vi "RT Main v0.61.vi"() -> ()   [LabVIEW 2017]
uses:
  support/Controls/All Inputs.ctl
  support/Controls/Index Details.ctl
  Controls/Auto Delays.ctl
  Global Variables/RT GV.vi
  Global Variables/FPGA GV.vi
  <vilib>/Utility/error.llb/Error Cluster From Error Code.vi
  <vilib>/rvi/errors/niLvFpgaAdjustHostInterfaceError.vi
  Global Variables/Network Globals.vi
  support/Message Queue/Enqueue Message (Single).vi
  <vilib>/FPGAPlugInAG/Dynamic/niLvFpga_Close_Dynamic.vi
  <vilib>/rvi/interface/nirviReadWriteControl/nirviReadWriteControl.xnode
  Controls/FPGA Ref.ctl
  <vilib>/rvi/interface/nirviCloseFPGA/nirviCloseFPGA.xnode
  support/Message Queue/Message Queue.lvlib
  NiFpgaLv.dll
  <vilib>/rvi/interface/Simulation/niFpgaSimulationCallBeginRW.vi
panel:
  in  "Stop Button 2":bool
  out "Agitator Delays":u32[](array[numeric])=[400, 5000]
  out "error out":errorcluster
  out "Wrong Message":string
  in  "Stop Button":bool
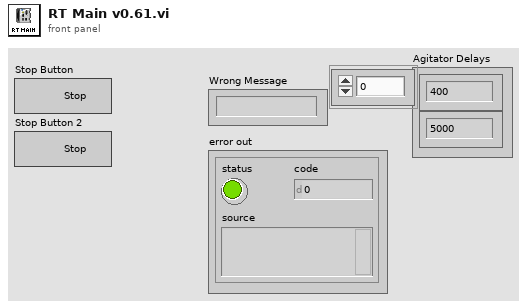
[diagram p1: front panel]
types:
  T1 = typedef "FPGA Ref.ctl" = refnum<k20>
  T2 = cluster{"TL_Red":bool, "TL_Orange":bool, "TL_Green":bool, "TL_Buzzer":bool, "SOL_Index_Rotary_CW":bool, "SOL_Index_CNVR_Rotary_CCW":bool, "SOL_Index_CNVR_Stopper_Rear":bool, "SOL_Index_CNVR_Output _Separator _Rear":bool, "Bowl  Feeder_ ON":bool, "Pump_CNVR_Motor _ON":bool, "SOL_Gating_CYL_Rear":bool, "SOL_Tube_Feed_Agitatator":bool, "SOL_Tube_Feed_Gating_CYL":bool, "SOL_Insertion _CYL":bool, "SOL_Insertion_Clamp_CYL":bool, "SOL_Cutting_CYL":bool, "SOL_Cutting_Clamp_CYL":bool, "SOL_Insertion_Air_Nozzle":bool, "SOL_Measurement_CYL":bool, "SOL_Measure_Clamp_CYL":bool, "SOL_Rejection CYL_1":bool, "SOL_Rejection CYL_2":bool, "SOL_Rejection CYL_3":bool, "SOL_Rejection CYL_4":bool, "DO1.24":bool, "DO1.25":bool, "DO1.26":bool, "DO1.27":bool, "DO1.28":bool, "DO1.29":bool, "DO1.30":bool, "DO1.31":bool}
  T3 = typedef "All Inputs.ctl" = cluster{"DI 1":cluster{"Machine_ON":bool, "E_stop ":bool, "SW_Pressure":bool, "SW_Start ":bool, "SW_Reset":bool, "SW_Stop":bool, "SW_Door":bool, "RS_Index_Rotary_CW":bool, "RS_Index_Rotary_CCW":bool, "RS_Index_Stopper _Rear":bool, "RS_Index_Output_Separator_Rear":bool, "PES_Index_Pallet_Sensor":bool, "PES_Index_Output_Part Sensor":bool, "ICS_BF_Low_Level_1":bool, "ICS_BF_Low_Level_2":bool, "ICS_BF_Pump_CNVR_Full_1":bool, "ICS_BF_Pump_CNVR_Full_2":bool, "ICS_BF_Pump_CNVR_Full_3":bool, "ICS_BF_Pump_CNVR_Full_4":bool, "PES_PC_Pump Presence_1":bool, "PES_PC_Pump Presence_2":bool, "PES_PC_Pump Presence_3":bool, "PES_PC_Pump Presence_4":bool, "RS_PC_Gating_Front":bool, "PES_Pump_Interference":bool, "PES_TF_Low_Level":bool, "PES_Tube Presence_1":bool, "PES_Tube Presence_2":bool, "PES_Tube Presence_3":bool, "PES_Tube Presence_4":bool, "DI1.30":bool, "DI1.31":bool}, "DI 2":cluster{"RS_Agitatator_1_Rear ":bool, "RS_Agitatator_2_Rear ":bool, "RS_TF_Gating CYL_Rear":bool, "RS_Insertion_1_Rear":bool, "RS_Insertion_1_Front":bool, "RS_Insertion _2_Rear":bool, "RS_Insertion _2_Front":bool, "RS_Insertion _3_Rear":bool, "RS_Insertion _3_Front":bool, "RS_Insertion _4_Rear":bool, "RS_Insertion _4_Front":bool, "RS_Insertion_Clamp_Rear":bool, "RS_Cutting_Rear":bool, "RS_Cutting_Clamp _Rear":bool, "RS_Measurement_1_Rear":bool, "RS_Measurement_2_Rear":bool, "RS_Measurement_3_Rear":bool, "RS_Measurement_4_Rear":bool, "RS_Measure_Clamp_Rear":bool, "RS_Rejection_1_Rear":bool, "RS_Rejection_2_Rear":bool, "RS_Rejection_3_Rear":bool, "RS_Rejection_4_Rear":bool, "DI2.23":bool, "DI2.24":bool, "DI2.25":bool, "DI2.26":bool, "DI2.27":bool, "DI2.28":bool, "DI2.29":bool, "DI2.30":bool, "DI2.31":bool}, "IAS 1":dbl, "IAS 2":dbl, "IAS 3":dbl, "IAS 4":dbl, "DO 1":cluster{"TL_Red":bool, "TL_Orange":bool, "TL_Green":bool, "TL_Buzzer":bool, "SOL_Index_Rotary_CW":bool, "SOL_Index_CNVR_Rotary_CCW":bool, "SOL_Index_CNVR_Stopper_Rear":bool, "SOL_Index_CNVR_Output _Separator _Rear":bool, "Bowl  Feeder_ ON":bool, "Pump_CNVR_Motor _ON":bool, "SOL_PC_Gating_CYL_Rear":bool, "SOL_Tube_Feed_Agitatator":bool, "SOL_Tube_Feed_Gating_CYL":bool, "SOL_Insertion _CYL":bool, "SOL_Insertion_Clamp_CYL":bool, "SOL_Cutting_CYL":bool, "SOL_Cutting_Clamp_CYL":bool, "SOL_Insertion_Air_Nozzle":bool, "SOL_Measurement_CYL":bool, "SOL_Measure_Clamp_CYL":bool, "SOL_Rejection CYL_1":bool, "SOL_Rejection CYL_2":bool, "SOL_Rejection CYL_3":bool, "SOL_Rejection CYL_4":bool, "DO1.24":bool, "DO1.25":bool, "DO1.26":bool, "DO1.27":bool, "DO1.28":bool, "DO1.29":bool, "DO1.30":bool, "DO1.31":bool}}
  T4 = typedef "Index Details.ctl" = cluster{"Time (ms)":u32, "Waveform Graph":i16[]}
  T5 = typedef "Auto Delays.ctl" = cluster{"Agitator Delays":u32[], "TF Delays":u32[], "Insertion Delays":u32[], "Cutting Delays":u32[], "PF Delays":u32[], "Measur. Delays":u32[], "Reject Delays":u32[]}
  T6 = cluster{T5, "Reject Pallets":cluster{"Reject 1":bool, "Reject 2":bool, "Reject 3":bool, "Reject 4":bool}}
  T7 = cluster{"TL_Red":bool, "TL_Orange":bool, "TL_Green":bool, "TL_Buzzer":bool, "SOL_Index_Rotary_CW":bool, "SOL_Index_CNVR_Rotary_CCW":bool, "SOL_Index_CNVR_Stopper_Rear":bool, "SOL_Index_CNVR_Output _Separator _Rear":bool, "Bowl  Feeder_ ON":bool, "Pump_CNVR_Motor _ON":bool, "SOL_PC_Gating_CYL_Rear":bool, "SOL_Tube_Feed_Agitatator":bool, "SOL_Tube_Feed_Gating_CYL":bool, "SOL_Insertion _CYL":bool, "SOL_Insertion_Clamp_CYL":bool, "SOL_Cutting_CYL":bool, "SOL_Cutting_Clamp_CYL":bool, "SOL_Insertion_Air_Nozzle":bool, "SOL_Measurement_CYL":bool, "SOL_Measure_Clamp_CYL":bool, "SOL_Rejection CYL_1":bool, "SOL_Rejection CYL_2":bool, "SOL_Rejection CYL_3":bool, "SOL_Rejection CYL_4":bool, "DO1.24":bool, "DO1.25":bool, "DO1.26":bool, "DO1.27":bool, "DO1.28":bool, "DO1.29":bool, "DO1.30":bool, "DO1.31":bool}
  T8 = cluster{"Machine_ON":bool, "E_stop ":bool, "SW_Pressure":bool, "SW_Start ":bool, "SW_Reset":bool, "SW_Stop":bool, "SW_Door":bool, "RS_Index_Rotary_CW":bool, "RS_Index_Rotary_CCW":bool, "RS_Index_Stopper _Rear":bool, "RS_Index_Output_Separator_Rear":bool, "PES_Index_Pallet_Sensor":bool, "PES_Index_Output_Part Sensor":bool, "ICS_BF_Low_Level_1":bool, "ICS_BF_Low_Level_2":bool, "ICS_BF_Pump_CNVR_Full_1":bool, "ICS_BF_Pump_CNVR_Full_2":bool, "ICS_BF_Pump_CNVR_Full_3":bool, "ICS_BF_Pump_CNVR_Full_4":bool, "PES_PC_Pump Presence_1":bool, "PES_PC_Pump Presence_2":bool, "PES_PC_Pump Presence_3":bool, "PES_PC_Pump Presence_4":bool, "RS_PC_Gating_Front":bool, "PES_Pump_Interference":bool, "PES_TF_Low_Level":bool, "PES_Tube Presence_1":bool, "PES_Tube Presence_2":bool, "PES_Tube Presence_3":bool, "PES_Tube Presence_4":bool, "DI1.30":bool, "DI1.31":bool}
  T9 = cluster{"RS_Agitatator_1_Rear ":bool, "RS_Agitatator_2_Rear ":bool, "RS_TF_Gating CYL_Rear":bool, "RS_Insertion_1_Rear":bool, "RS_Insertion_1_Front":bool, "RS_Insertion _2_Rear":bool, "RS_Insertion _2_Front":bool, "RS_Insertion _3_Rear":bool, "RS_Insertion _3_Front":bool, "RS_Insertion _4_Rear":bool, "RS_Insertion _4_Front":bool, "RS_Insertion_Clamp_Rear":bool, "RS_Cutting_Rear":bool, "RS_Cutting_Clamp _Rear":bool, "RS_Measurement_1_Rear":bool, "RS_Measurement_2_Rear":bool, "RS_Measurement_3_Rear":bool, "RS_Measurement_4_Rear":bool, "DI2.18":bool, "RS_Rejection_1_Rear":bool, "RS_Rejection_2_Rear":bool, "RS_Rejection_3_Rear":bool, "RS_Rejection_4_Rear":bool, "DI2.23":bool, "DI2.24":bool, "DI2.25":bool, "DI2.26":bool, "DI2.27":bool, "DI2.28":bool, "DI2.29":bool, "DI2.30":bool, "DI2.31":bool}
  T10 = cluster{"Reject 1":bool, "Reject 2":bool, "Reject 3":bool, "Reject 4":bool}
  T11 = typedef "Auto Times.ctl" = cluster{"Index Time":u32, "TF Time":u32, "Insertion Time":u32, "Cutting Time":u32, "PF Time":u32, "Meas. Time":u32, "Reject Time":u32}
  T12 = cluster{"Auto Times":T11, "Measurements":cluster{"1":dbl, "2":dbl, "3":dbl, "4":dbl}, "OutputCount":u32, "error out":errorcluster}
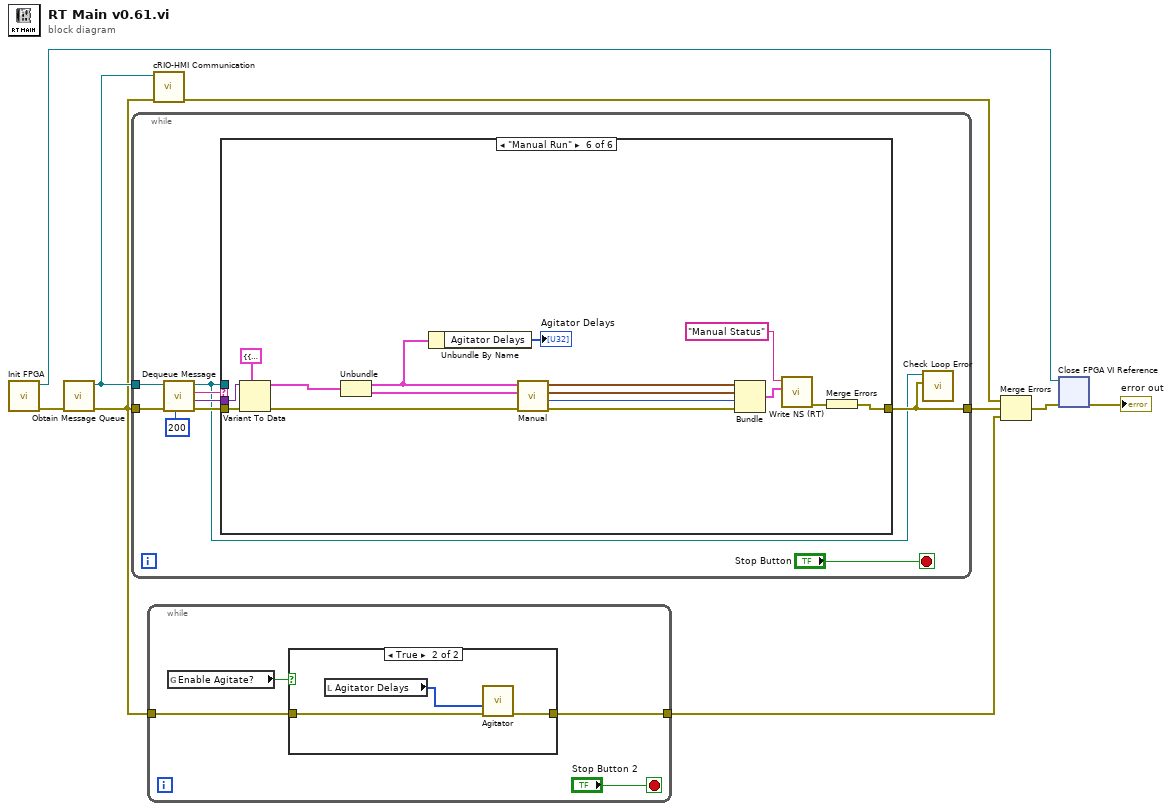
[diagram p0: block diagram]
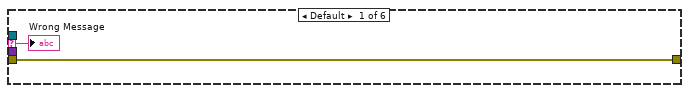
[diagram p3: hidden frame]
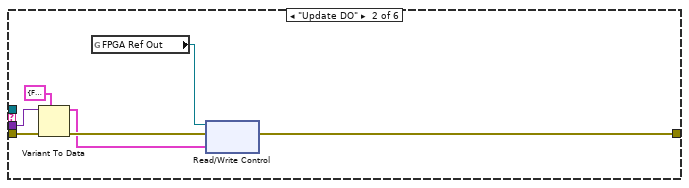
[diagram p4: hidden frame]
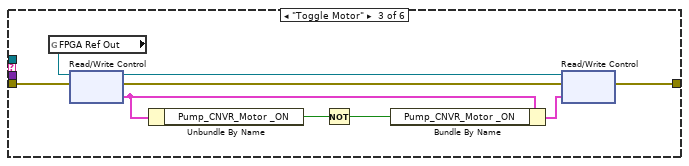
[diagram p5: hidden frame]
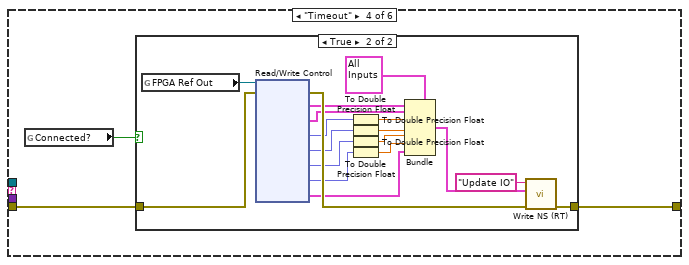
[diagram p6: hidden frame]
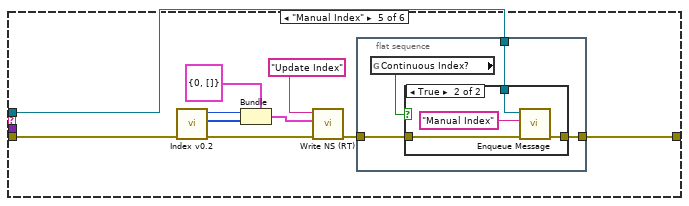
[diagram p8: hidden frame]
diagram:
  n1 = call "Init FPGA.vi"() -> ("error out"=w9:errorcluster, "FPGA Ref Out"=w3:T1)  [unwired: 10 in]
  n2 = call "Obtain Message Queue.vi"("error in (no error)"=w9) -> ("error out"=w2:errorcluster, "Message Queue"=w8:refnum<queue>)  [unwired: 9 in]
  n3 = while {
    tunnel: w2 -> [w17]
    tunnel: w8 -> [w16]
    tunnel: [w12] -> w7
    stop <- "Stop Button" stop-if-true
    n4 = call "Dequeue Message.vi"("timeout"=200, "error in (no error)"=w17, "Message Queue"=w16) -> ("error out"=w15:errorcluster, "Message Data"=w13:variant, "Message"=w14:string, "dup Message Queue"=w11:refnum<queue>)  [unwired: 5 in]
    n5 = case shown="\"Manual Run\"" w14 {
      selector: w14 -> [w20 _ _ _ _ _]
      tunnel: w15 -> [w19 w27 w35 w38 w68 w93]
      tunnel: w11 -> [_ _ _ _ w60 _]
      tunnel: w13 -> [_ w26 _ _ _ w92]
      tunnel: [w19 w22 w33 w39 w61 w88] -> w12
      frame Default {
        "Wrong Message" <- w20
      }
      frame "Update DO" {
        n6 = Variant To Data(error in=w27, type=T2 {"TL_Red"=FALSE, "TL_Orange"=FALSE, "TL_Green"=FALSE, "TL_Buzzer"=FALSE, "SOL_Index_Rotary_CW"=FALSE, "SOL_Index_CNVR_Rotary_CCW"=FALSE, "SOL_Index_CNVR_Stopper_Rear"=FALSE, "SOL_Index_CNVR_Output _Separator _Rear"=FALSE, "Bowl  Feeder_ ON"=FALSE, "Pump_CNVR_Motor _ON"=FALSE, "SOL_Gating_CYL_Rear"=FALSE, "SOL_Tube_Feed_Agitatator"=FALSE, "SOL_Tube_Feed_Gating_CYL"=FALSE, "SOL_Insertion _CYL"=FALSE, "SOL_Insertion_Clamp_CYL"=FALSE, "SOL_Cutting_CYL"=FALSE, "SOL_Cutting_Clamp_CYL"=FALSE, "SOL_Insertion_Air_Nozzle"=FALSE, "SOL_Measurement_CYL"=FALSE, "SOL_Measure_Clamp_CYL"=FALSE, "SOL_Rejection CYL_1"=FALSE, "SOL_Rejection CYL_2"=FALSE, "SOL_Rejection CYL_3"=FALSE, "SOL_Rejection CYL_4"=FALSE, "DO1.24"=FALSE, "DO1.25"=FALSE, "DO1.26"=FALSE, "DO1.27"=FALSE, "DO1.28"=FALSE, "DO1.29"=FALSE, "DO1.30"=FALSE, "DO1.31"=FALSE} ("DO 1"), Variant=w26) -> (data=w21:T2, error out=w23:errorcluster)
        n7 = global read "FPGA GV.vi" "FPGA Ref Out"() -> (w24:T1)
        n8 = xnode "Read/Write Control"("FPGA VI Reference In"=w24, "error in"=w23, "DO 1"=w21) -> ("error out"=w22:errorcluster)  [unwired: 1 out]
      }
      frame "Toggle Motor" {
        n9 = global read "FPGA GV.vi" "FPGA Ref Out"() -> (w36:T1)
        n10 = xnode "Read/Write Control"("FPGA VI Reference In"=w36, "error in"=w35) -> ("FPGA VI Reference Out"=w32:T1, "error out"=w34:errorcluster, "DO 1"=w30:T7)
        n11 = Unbundle By Name(w30) -> ("Pump_CNVR_Motor _ON"=w31:bool)
        n12 = Not(x=w31) -> (.not. x?=w28:bool)
        n13 = Bundle By Name(cluster=w30, "Pump_CNVR_Motor _ON"=w28) -> (w29:T7)
        n14 = xnode "Read/Write Control"("FPGA VI Reference In"=w32, "error in"=w34, "DO 1"=w29) -> ("error out"=w33:errorcluster)  [unwired: 1 out]
      }
      frame "Timeout" {
        n15 = global read "Network Globals.vi" "Connected?"() -> (w37:bool)
        n16 = case shown="True" w37 {
          tunnel: [w40 w57] -> w39
          tunnel: w38 -> [w40 w55]
          frame False {
          }
          frame True {
            n17 = global read "FPGA GV.vi" "FPGA Ref Out"() -> (w56:T1)
            n18 = xnode "Read/Write Control"("FPGA VI Reference In"=w56, "error in"=w55) -> ("error out"=w54:errorcluster, "DI 1"=w53:T8, "DI 2"=w52:T9, "AI0"=w51:fxp<+/-,27,6>, "AI1"=w46:fxp<+/-,27,6>, "AI2"=w45:fxp<+/-,27,6>, "AI3"=w44:fxp<+/-,27,6>, "DO 1"=w41:T7)  [unwired: 1 out]
            n19 = To Double Precision Float(number=w51) -> (double precision float=w50:dbl)
            n20 = To Double Precision Float(number=w46) -> (double precision float=w49:dbl)
            n21 = To Double Precision Float(number=w45) -> (double precision float=w48:dbl)
            n22 = To Double Precision Float(number=w44) -> (double precision float=w47:dbl)
            n23 = Bundle(cluster=T3 {"DI 1"={"Machine_ON"=FALSE, "E_stop "=FALSE, "SW_Pressure"=FALSE, "SW_Start "=FALSE, "SW_Reset"=FALSE, "SW_Stop"=FALSE, "SW_Door"=FALSE, "RS_Index_Rotary_CW"=FALSE, "RS_Index_Rotary_CCW"=FALSE, "RS_Index_Stopper _Rear"=FALSE, "RS_Index_Output_Separator_Rear"=FALSE, "PES_Index_Pallet_Sensor"=FALSE, "PES_Index_Output_Part Sensor"=FALSE, "ICS_BF_Low_Level_1"=FALSE, "ICS_BF_Low_Level_2"=FALSE, "ICS_BF_Pump_CNVR_Full_1"=FALSE, "ICS_BF_Pump_CNVR_Full_2"=FALSE, "ICS_BF_Pump_CNVR_Full_3"=FALSE, "ICS_BF_Pump_CNVR_Full_4"=FALSE, "PES_PC_Pump Presence_1"=FALSE, "PES_PC_Pump Presence_2"=FALSE, "PES_PC_Pump Presence_3"=FALSE, "PES_PC_Pump Presence_4"=FALSE, "RS_PC_Gating_Front"=FALSE, "PES_Pump_Interference"=FALSE, "PES_TF_Low_Level"=FALSE, "PES_Tube Presence_1"=FALSE, "PES_Tube Presence_2"=FALSE, "PES_Tube Presence_3"=FALSE, "PES_Tube Presence_4"=FALSE, "DI1.30"=FALSE, "DI1.31"=FALSE}, "DI 2"={"RS_Agitatator_1_Rear "=FALSE, "RS_Agitatator_2_Rear "=FALSE, "RS_TF_Gating CYL_Rear"=FALSE, "RS_Insertion_1_Rear"=FALSE, "RS_Insertion_1_Front"=FALSE, "RS_Insertion _2_Rear"=FALSE, "RS_Insertion _2_Front"=FALSE, "RS_Insertion _3_Rear"=FALSE, "RS_Insertion _3_Front"=FALSE, "RS_Insertion _4_Rear"=FALSE, "RS_Insertion _4_Front"=FALSE, "RS_Insertion_Clamp_Rear"=FALSE, "RS_Cutting_Rear"=FALSE, "RS_Cutting_Clamp _Rear"=FALSE, "RS_Measurement_1_Rear"=FALSE, "RS_Measurement_2_Rear"=FALSE, "RS_Measurement_3_Rear"=FALSE, "RS_Measurement_4_Rear"=FALSE, "RS_Measure_Clamp_Rear"=FALSE, "RS_Rejection_1_Rear"=FALSE, "RS_Rejection_2_Rear"=FALSE, "RS_Rejection_3_Rear"=FALSE, "RS_Rejection_4_Rear"=FALSE, "DI2.23"=FALSE, "DI2.24"=FALSE, "DI2.25"=FALSE, "DI2.26"=FALSE, "DI2.27"=FALSE, "DI2.28"=FALSE, "DI2.29"=FALSE, "DI2.30"=FALSE, "DI2.31"=FALSE}, "IAS 1"=0.0, "IAS 2"=0.0, "IAS 3"=0.0, "IAS 4"=0.0, "DO 1"={"TL_Red"=FALSE, "TL_Orange"=FALSE, "TL_Green"=FALSE, "TL_Buzzer"=FALSE, "SOL_Index_Rotary_CW"=FALSE, "SOL_Index_CNVR_Rotary_CCW"=FALSE, "SOL_Index_CNVR_Stopper_Rear"=FALSE, "SOL_Index_CNVR_Output _Separator _Rear"=FALSE, "Bowl  Feeder_ ON"=FALSE, "Pump_CNVR_Motor _ON"=FALSE, "SOL_PC_Gating_CYL_Rear"=FALSE, "SOL_Tube_Feed_Agitatator"=FALSE, "SOL_Tube_Feed_Gating_CYL"=FALSE, "SOL_Insertion _CYL"=FALSE, "SOL_Insertion_Clamp_CYL"=FALSE, "SOL_Cutting_CYL"=FALSE, "SOL_Cutting_Clamp_CYL"=FALSE, "SOL_Insertion_Air_Nozzle"=FALSE, "SOL_Measurement_CYL"=FALSE, "SOL_Measure_Clamp_CYL"=FALSE, "SOL_Rejection CYL_1"=FALSE, "SOL_Rejection CYL_2"=FALSE, "SOL_Rejection CYL_3"=FALSE, "SOL_Rejection CYL_4"=FALSE, "DO1.24"=FALSE, "DO1.25"=FALSE, "DO1.26"=FALSE, "DO1.27"=FALSE, "DO1.28"=FALSE, "DO1.29"=FALSE, "DO1.30"=FALSE, "DO1.31"=FALSE}}, "DI 1"=w53, "DI 2"=w52, "IAS 1"=w50, "IAS 2"=w49, "IAS 3"=w48, "IAS 4"=w47, "DO 1"=w41) -> (w43:T3)
            n24 = call "Write NS (RT).vi"("error in (no error)"=w54, "Message Data"=w43, "Message"="Update IO") -> ("error out"=w57:errorcluster)  [unwired: 8 in]
          }
        }
      }
      frame "Manual Index" {
        n25 = call "Index v0.2.vi"("error in (no error)"=w68) -> ("error out"=w66:errorcluster, "Waveform Graph"=w64:i16[], "Index Time"=w65:u32)  [unwired: 7 in, 1 out]
        n26 = Bundle(cluster=T4 {"Time (ms)"=0, "Waveform Graph"=[]}, "Time (ms)"=w65, "Waveform Graph"=w64) -> (w63:T4)
        n27 = call "Write NS (RT).vi"("error in (no error)"=w66, "Message Data"=w63, "Message"="Update Index") -> ("error out"=w62:errorcluster)  [unwired: 8 in]
        n28 = flat-sequence {
          tunnel: w62 -> [w72]
          tunnel: [w71] -> w61
          tunnel: w60 -> [w69]
          frame #0 {
            n29 = global read "RT GV.vi" "Continuous Index?"() -> (w70:bool)
            n30 = case shown="True" w70 {
              tunnel: w72 -> [w73 w77]
              tunnel: [w73 w76] -> w71
              tunnel: w69 -> [_ w74]
              frame False {
              }
              frame True {
                n31 = call-poly "Enqueue Message.vi"("error in (no error)"=w77, "Message"="Manual Index", "Message Queue"=w74) -> ("error out"=w76:errorcluster)  [unwired: 7 in, 1 out]
              }
            }
          }
        }
      }
      frame "Manual Run" {
        n32 = Variant To Data(error in=w93, type=T6 {{"Agitator Delays"=[1000], "TF Delays"=[1000], "Insertion Delays"=[1000], "Cutting Delays"=[1000], "PF Delays"=[1000], "Measur. Delays"=[1000], "Reject Delays"=[1000]}, "Reject Pallets"={"Reject 1"=FALSE, "Reject 2"=FALSE, "Reject 3"=FALSE, "Reject 4"=FALSE}}, Variant=w92) -> (data=w83:T6, error out=w91:errorcluster)
        n33 = Unbundle(w83) -> (w79:T5, "Reject Pallets"=w82:T10)
        n34 = Unbundle By Name(w79) -> ("Agitator Delays"=→"Agitator Delays":u32[])
        n35 = call "Manual.vi"("error in (no error)"=w91, "Reject Pallets"=w82, "Auto Delays"=w79) -> ("error out"=w81:errorcluster, "OutputCount"=w80:u32, "Measurements"=w85:cluster{"1":dbl, "2":dbl, "3":dbl, "4":dbl}, "Auto Times"=w87:T11)  [unwired: 5 in]
        n36 = Bundle("Auto Times"=w87, "Measurements"=w85, "OutputCount"=w80, "error out"=w81) -> (w86:T12)  [unwired: 1 in]
        n37 = call "Write NS (RT).vi"("Message Data"=w86, "Message"="Manual Status") -> ("error out"=w89:errorcluster)  [unwired: 9 in]
        n38 = Merge Errors(w89) -> (w88:errorcluster)
      }
    }
    n39 = call "Check Loop Error.vi"("error to process"=w12, "Message Queue"=w11) -> ()  [unwired: 8 in, 2 out]
  }
  n40 = while {
    tunnel: w2 -> [w97]
    tunnel: [w94] -> w1
    stop <- "Stop Button 2" stop-if-true
    n41 = global read "RT GV.vi" "Enable Agitate?"() -> (w96:bool)
    n42 = case shown="True" w96 {
      tunnel: w97 -> [w98 w101]
      tunnel: [w98 w99] -> w94
      frame False {
      }
      frame True {
        n43 = local read "Agitator Delays"() -> (w100:u32[])
        n44 = call "Agitator.vi"("error in (no error)"=w101, "Agitator Delays"=w100) -> ("error out"=w99:errorcluster)  [unwired: 8 in, 1 out]
      }
    }
  }
  n45 = call "cRIO-HMI Communication.vi"("error in (no error)"=w2, "Message Queue"=w8) -> ("error out"=w6:errorcluster)  [unwired: 9 in]
  n46 = Merge Errors(w6, w7, w1) -> (w5:errorcluster)
  n47 = xnode ("Close FPGA VI Reference")("FPGA VI Reference In"=w3, "error in"=w5) -> ("error out"=→"error out":errorcluster)
